vi "setFormat.vi"(8 "error in (no error)":errorcluster, 10 "format":T1, 11 "Instrument.VSource in":refnum<class "Instrument.VNA.lvclass">) -> (0 "error out":errorcluster, 3 "Instrument.VSource out":refnum<class "Instrument.VNA.lvclass">)   [LabVIEW 2019, in "Instrument.VNA.lvclass"]
uses:
  Instrument.VNA.lvclass
  C:/Users/patrick/Documents/GitHub/Instrument-Framework/lvsrc/Instrument/Instrument.lvclass
  Typedefs/Format--enum.ctl
  facca5f9-ceb2-4251-b21f-2fede6c04c13.vi
  facca5f9-ceb2-4251-b21f-2fede6c04c13.vi/a25e8f9e-1138-41ff-8e7b-f964a31040b1.vi
  facca5f9-ceb2-4251-b21f-2fede6c04c13.vi/a25e8f9e-1138-41ff-8e7b-f964a31040b1.vi/71e6bf62-da74-425d-8a32-d5a7942c0589.vi
  facca5f9-ceb2-4251-b21f-2fede6c04c13.vi/a25e8f9e-1138-41ff-8e7b-f964a31040b1.vi/8b8705b8-81c1-4c8c-87b4-e60c314c5c3e.vi
  Instrument/Private/Get RC Connection Status.vi
  Instrument/API/Send and Receive.vi
  <vilib>/Utility/Data Type/Get Type Information.vi
  <vilib>/JDP Science/JSONtext/JSON text to Variant.vi
  <vilib>/JDP Science/JSONtext/LVClass Serializer/JSONtext LVClass Serializer.lvclass
  Instrument/Instrument.lvclass
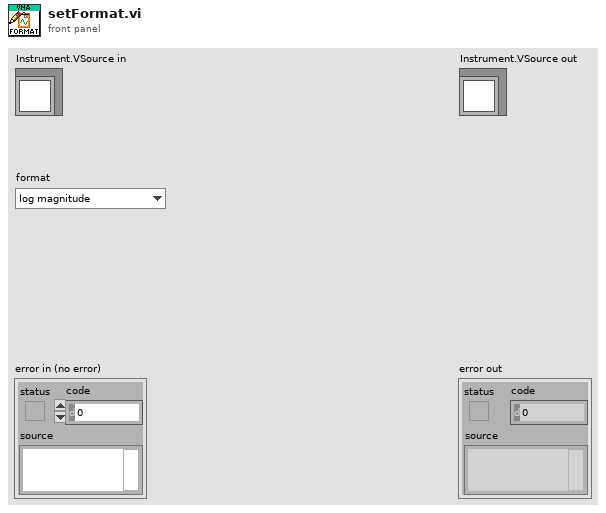
[diagram p1: front panel]
types:
  T1 = typedef "Instrument.VNA.lvclass/Format--enum.ctl" = enum16{"log magnitude", "phase", "delay", "Smith chart", "polar", "linear magnitude", "standing wave ratio", "real", "imaginary"}
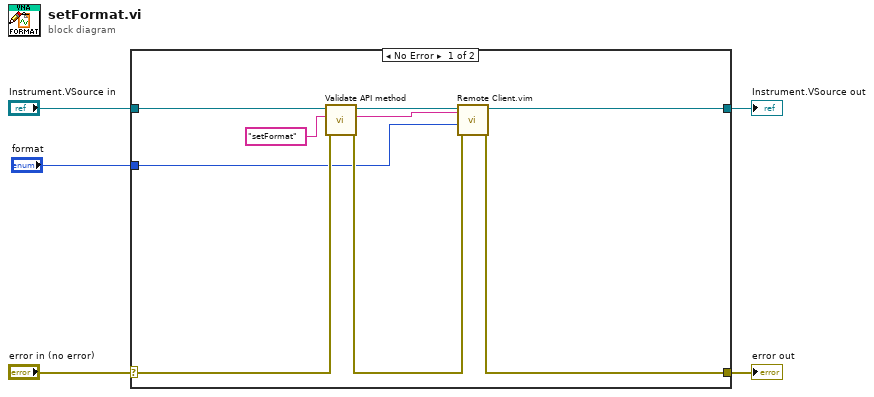
[diagram p0: block diagram]
diagram:
  n1 = case shown="No Error" "error in (no error)" {
    selector: "error in (no error)" -> [w9 w16]
    tunnel: [w8 w16] -> w4
    tunnel: [w11 w15] -> w2
    tunnel: "Instrument.VSource in" -> [w12 w15]
    tunnel: "format" -> [w7 _]
    frame No Error {
      n2 = call "Validate API method.vi"("error in (no error)"=w9, "Command in"="setFormat" ("error message (\"\")"), "Instrument in"=w12) -> ("error out"=w10:errorcluster, "command out"=w6:string, "Instrument out"=w13:refnum<class "Instrument.VNA.lvclass">)  [unwired: 6 in]
      n3 = call "Remote Client.vim"("Data Out type"=w6, "error in (no error)"=w10, "Data in"=w7, "Instrument in"=w13) -> ("error out"=w8:errorcluster, "Instrument out"=w11:refnum<class "Instrument.VNA.lvclass">)  [unwired: 4 in, 2 out]
    }
    frame Error {
    }
  }
  "error out" <- w4
  "Instrument.VSource out" <- w2
